vi "Controle_da_mesa_v3.vi"() -> ()   [LabVIEW 2017]
uses:
  <vilib>/Platform/TimedLoop/XDataNode/XDataNode.xnode
  <vilib>/Platform/TimedLoop/XDataNode/nitl_modes.ctl
  <vilib>/Platform/TimedLoop/XDataNode/XDNodeRunTimeDep.lvlib
  <vilib>/Platform/TimedLoop/XDataNode/wakeup.ctl
  <vilib>/Platform/TimedLoop/XDataNode/timing_clust.ctl
  <vilib>/Analysis/Matrix/NI_Matrix.lvlib
  <vilib>/Analysis/NI_AALPro.lvlib
  <vilib>/Analysis/NI_AALBase.lvlib
  <vilib>/Analysis/baseanly.llb/Real A x B.vi
  <vilib>/Analysis/Matrix/Numeric/Conversions/Matrix To Array - RM.vi
  <vilib>/Analysis/Matrix/Numeric/Conversions/Array To Matrix - RA.vi
  <vilib>/Analysis/Matrix/Numeric/Conversions/Array To Matrix - RA2.vi
  <vilib>/Analysis/_algsub.llb/Real PseudoInverse Matrix.vi
  <vilib>/rvi/interface/nirviCloseFPGA/nirviCloseFPGA.xnode
  <vilib>/rvi/interface/nirviMethod/nirviMethod.xnode
  <vilib>/rvi/interface/nirviMethod/StockFPGA_InlinedMethodWaitForSingleIRQ.vi
  <vilib>/FPGAPlugInAG/Dynamic/niLvFpga_WaitOnIrq_Dynamic.vi
  <vilib>/FPGAPlugInAG/Dynamic/niLvFpga_ReadFifo_Dynamic.vi
  <vilib>/rvi/errors/niLvFpgaMergeErrorWithErrorCode.vi
  <vilib>/FPGAPlugInAG/Dynamic/niLvFpga_AcknowledgeIrq_Dynamic.vi
  <vilib>/FPGAPlugInAG/Dynamic/niLvFpga_Close_Dynamic.vi
panel:
  out "Iteration Duration 2":i64
  out "error out 2":errorcluster
  out "error out":errorcluster
  in  "Stop_RT":bool
  out "Iteration Duration":i64
  out "INS":cluster{dbl[], sgl[]}[](graph)
  out "INS_R":bool
  out "CRC?":bool
  out "CRC Out":u16 format="%.0x"
  out "CRC_Input":u16 format="%x"
  out "LPI-X_R":sgl(slide)=-2.8742945e-05 scale=-6.0..6.0
  out "LPI-Y_R":sgl(slide)=-2.8742945e-05 scale=-6.0..6.0
  out "LPI-Z_R":sgl(slide)=-2.8742945e-05 scale=-6.0..6.0
  out "Longitude_R":sgl(slide)=-2.8742945e-05 scale=-180.0..180.0
  out "Altitude_R":sgl(slide)=-2.8742945e-05 scale=0.0..500.0
  out "Latitude_R":sgl(slide)=-2.8742945e-05 scale=-90.0..90.0
  out "Z_Accel_R":sgl(slide)=-2.8742945e-05 scale=-200.0..200.0
  out "X_Accel_R":sgl(slide)=-2.8742945e-05 scale=-200.0..200.0
  out "Y_Accel_R":sgl(slide)=-2.8742945e-05 scale=-200.0..200.0
  out "Z_Rate_R":sgl(slide)=-2.8742945e-05 scale=-300.0..300.0
  out "Y_ Rate_R":sgl(slide)=-2.8742945e-05 scale=-300.0..300.0
  out "X_Rate _R":sgl(slide)=-2.8742945e-05 scale=-300.0..300.0
  out "Yaw_R":sgl(slide)=-2.8742945e-05 scale=-180.0..180.0
  out "Pitch_R":sgl(slide)=-2.8742945e-05 scale=-90.0..90.0
  out "Roll_R":sgl(slide)=-2.8742945e-05 scale=-180.0..180.0
  out "Data Validity Time":u16[](array[numeric])
  out "Read String":string
  out "reserved 14":bool
  out "reserved 15":bool
  out "GC restarted 2":bool
  out "reserved 16":bool
  out "Init Align. M_Comp 2":bool
  out "Tick_Counter 2":u16
  out "Align_Word_Byte":bool[](array[boolean])
  out "GC_Counter 2":u32
  out "GC Align Counter (s) 2":bool[](array[boolean])
  out "Opp_Mode 2":string
  out "Fault_Code_HW 2":string
  out "ASE warning   2":bool
  out "Power warning 2":bool
  out "Motion Detection 2":bool
  out "RESERVED 4":bool
  out "RESERVED 5":bool
  out "RESERVED 6":bool
  out "Fault_Code 2":bool[](array[boolean])
  out "Operative_Mode 2":bool[](array[boolean])
  out "Op_Word_Byte":bool[](array[boolean])
  out "CRC_MSB 2":u8
  out "CRC_LSB 2":u8
  out "Status_Word_Byte":bool[](array[boolean])
  out "Data_Validity_Byte":bool[](array[boolean])
  out "outer previsto":dbl
  out "inner previsto":dbl
  in  "passo de predição":dbl=0.03 format="%#_13g"
  out "middle previsto":dbl
  out "Period":i64
  out "Middle":cluster{dbl[], dbl[]}[](graph)
  in  "Inicia seno":bool
  in  "Inner ON":bool
  in  "Middle ON":bool
  in  "Outer ON":bool
  in  "Amplitude Inner [deg]":dbl=1.0 format="%#_13g"
  in  "Amplitude Middle [deg]":dbl=1.0 format="%#_13g"
  in  "Amplitude Outer [deg]":dbl=1.0 format="%#_13g"
  in  "f inner [Hz]":dbl=1.0 format="%#_13g"
  in  "f middle [Hz]":dbl=1.0 format="%#_13g"
  in  "f outer [Hz]":dbl=1.0 format="%#_13g"
  out "spreadsheet string":string
  in  "UTC format":bool
  out "appended path":path
  out "concatenated string":string
  out "ACCEL":cluster{dbl, dbl, dbl} {"?" format="%1_6g"}
  out "RATE":cluster{dbl, dbl, dbl} {"?" format="%1_6g"}
  out "POS":cluster{dbl, dbl, dbl} {"?" format="%_6g"; "?" format="%#1_6g"}
  out "Tempo (s)":dbl
  out "string enviada para acutrol":string
  in  "Remote Host":string="192.168.53.1"
  in  "Para Controle da mesa":bool
  # "Atentar-se para que a posição inicial da mesa seja a mesma posição comandada. (Condições iniciais - Pos/Rate/Accel)"
  # "Monitor"
  # "Inner"
  # "Middle"
  # "Outer"
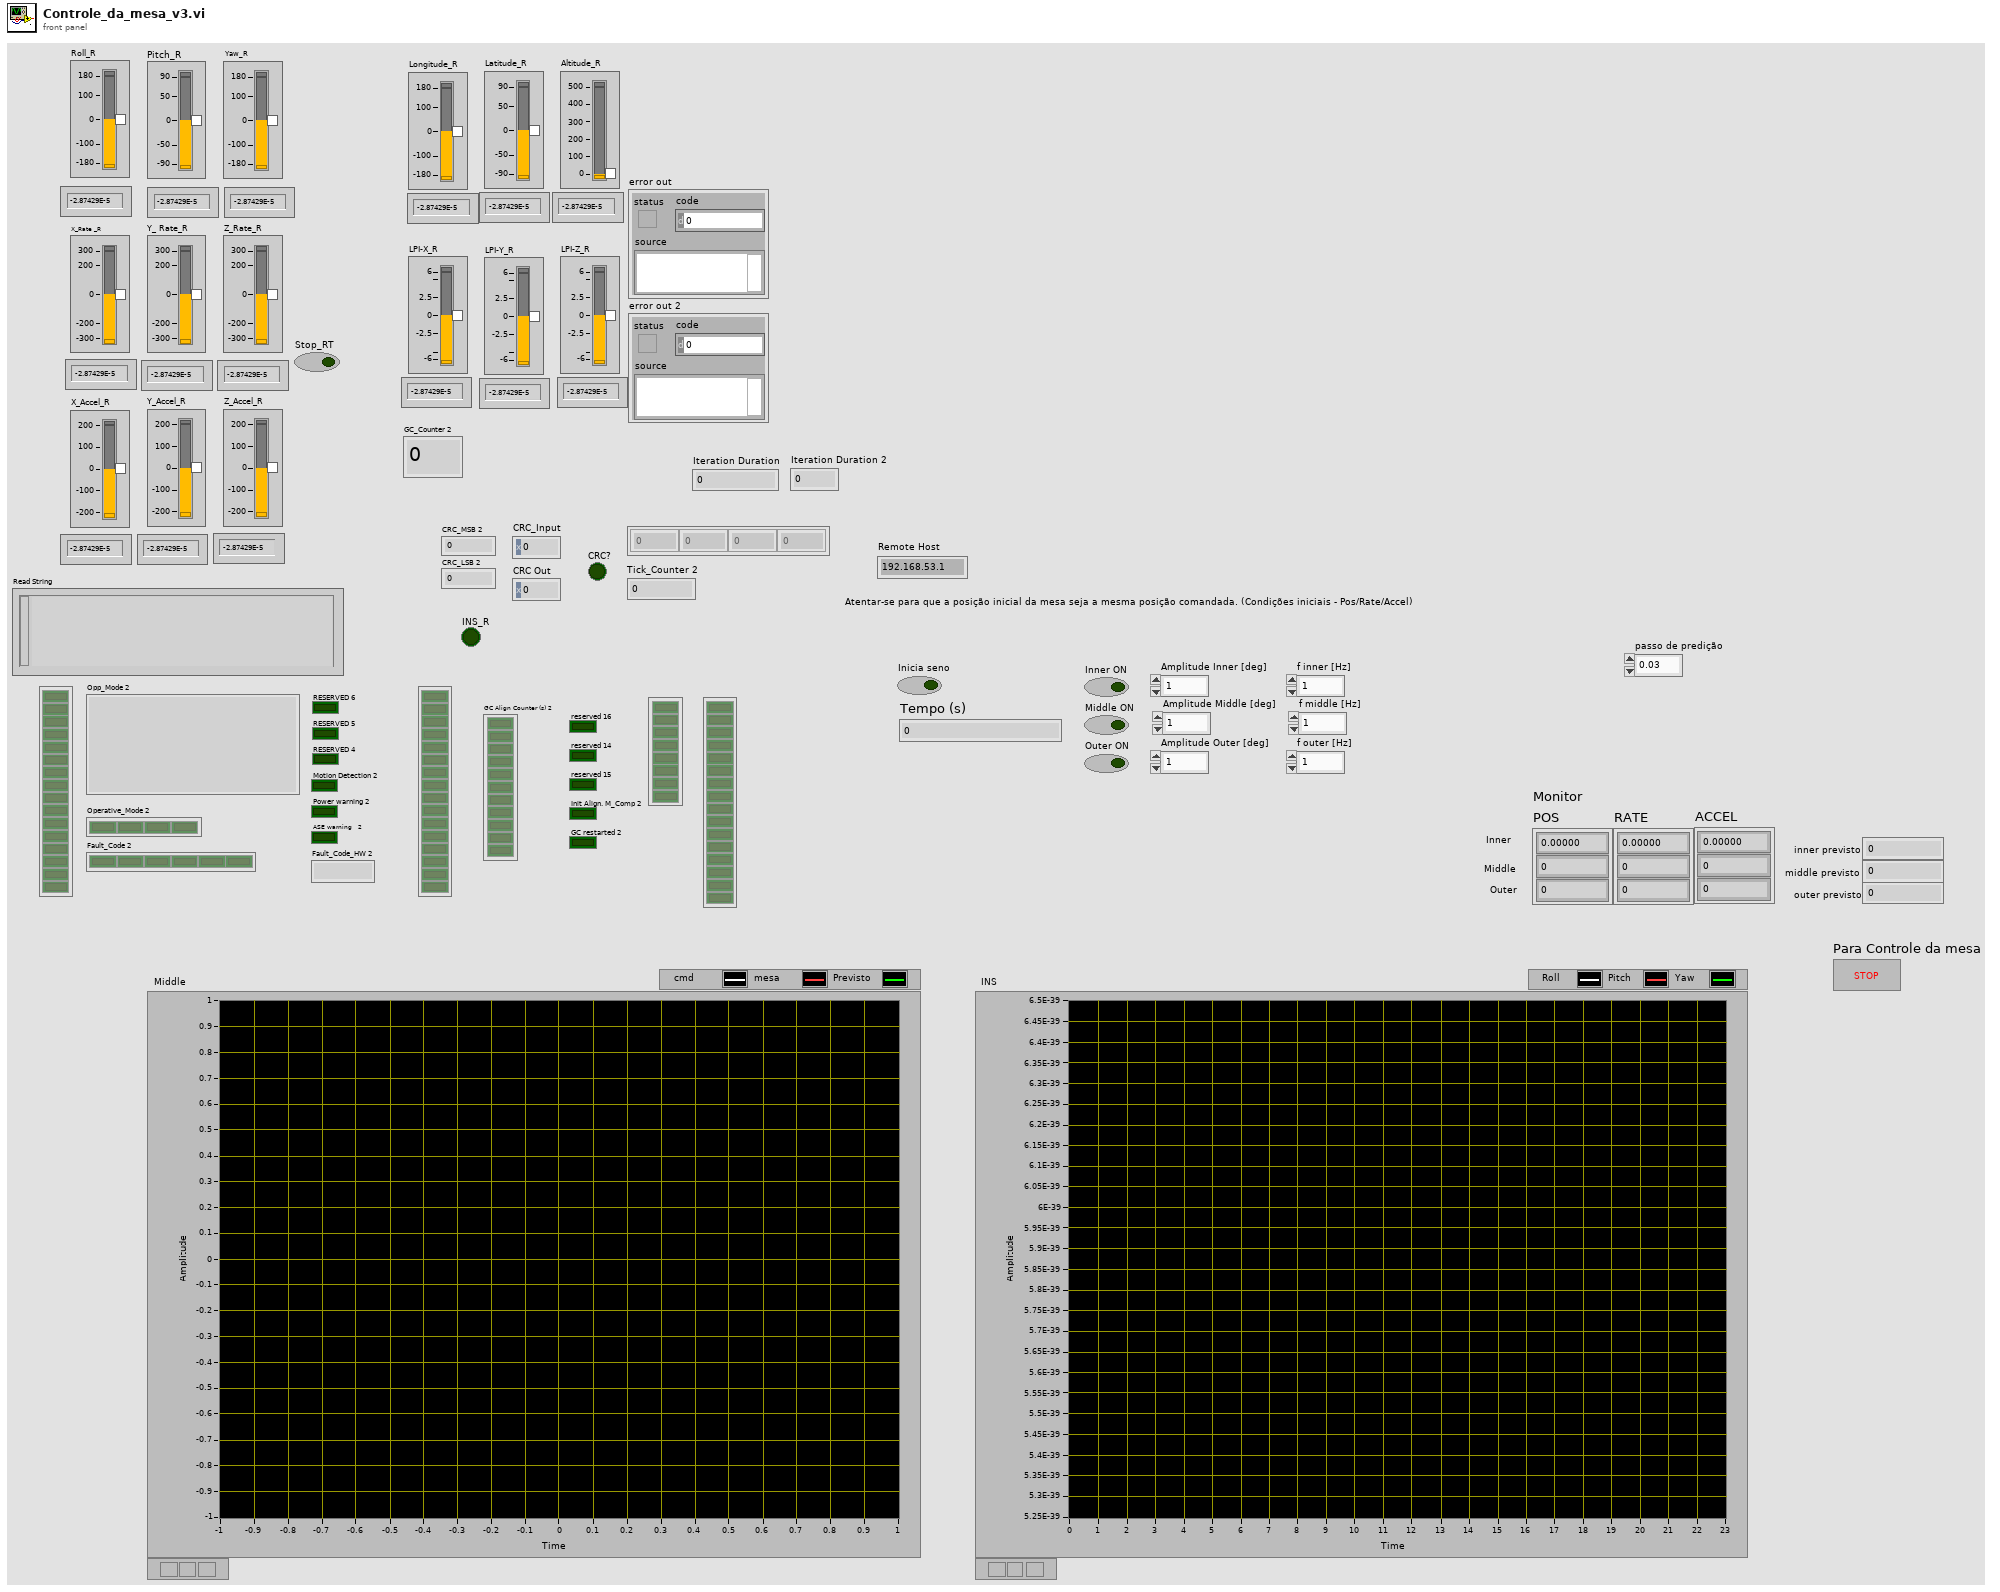
[diagram p1: front panel]
types:
  T1 = enum16{"open", "replace", "create", "open or create", "replace or create", "replace or create with confirmation"}
  T2 = typedef "XDNodeRunTimeDep.lvlib/timing_clust.ctl" = cluster{"Expected End [f-1]":u64, "Actual End [f-1]":u64, "Finished Late? [f-1]":bool, "Expected End [i-1]":u64, "Actual End [i-1]":u64, "Finished Late? [i-1]":bool, "Expected Start [i]":u64, "Actual Start [i]":u64, "Expected Start [f]":u64, "Actual Start [f]":u64, "Source Name":string, "Structure Name":string, "Period":i64, "Deadline":i64, "Offset":i64, "Start":i64, "Priority":i32, "Timeout":i32, "Mode":T3, "Wakeup Reason":T4, "Error":errorcluster, "Source Type":string, "Secondary Source Type":string, "Global End Time":u64, "Global Start Time":u64, "Frame Duration":u64, "Iteration Duration":u64, "Assigned CPU":i32, "I/O Scan Engine Mode":u32}
  T3 = typedef "XDNodeRunTimeDep.lvlib/nitl_modes.ctl" = enum32{"No Change", "Process missed periods, maintain original phase", "Discard missed periods, maintain original phase", "Process missed periods, ignore original phase", "Discard missed periods, ignore original phase"}
  T4 = typedef "XDNodeRunTimeDep.lvlib/wakeup.ctl" = enum32{"Normal", "Aborted", "Asynchronous wakeup", "Timing source error", "Timed loop error", "Timeout"}
  T5 = typedef "NI_Matrix.lvlib/RealMatrix.ctl" = dbl[][]
  T6 = cluster{"Roll_":sgl, "Pitch_":sgl, "Yaw_":sgl, "X_Rate":sgl, "Y_ Rate":sgl, "Z_Rate":sgl, "X_Accel":sgl, "Y_Accel":sgl, "Z_Accel":sgl, "Longitude":sgl, "Latitude":sgl, "Altitude":sgl, "LPI-X":sgl, "LPI-Y":sgl, "LPI-Z":sgl}
  T7 = cluster{"Op_Word_Byte":bool[], "Opp_Mode":string, "Operative_Mode":bool[], "RESERVED":bool, "RESERVED":bool, "RESERVED":bool, "Motion Detection":bool, "Power Warning":bool, "ASE Warning":bool, "Fault_Code":bool[], "Fault_Code_HW":string}
  T8 = cluster{"Align_Word_Byte":bool[], "GC Align Counter (s)":bool[], "GC_Counter":u32, "reserved":bool, "reserved":bool, "reserved":bool, "Init Align. M_Comp":bool, "GC restarted ":bool}
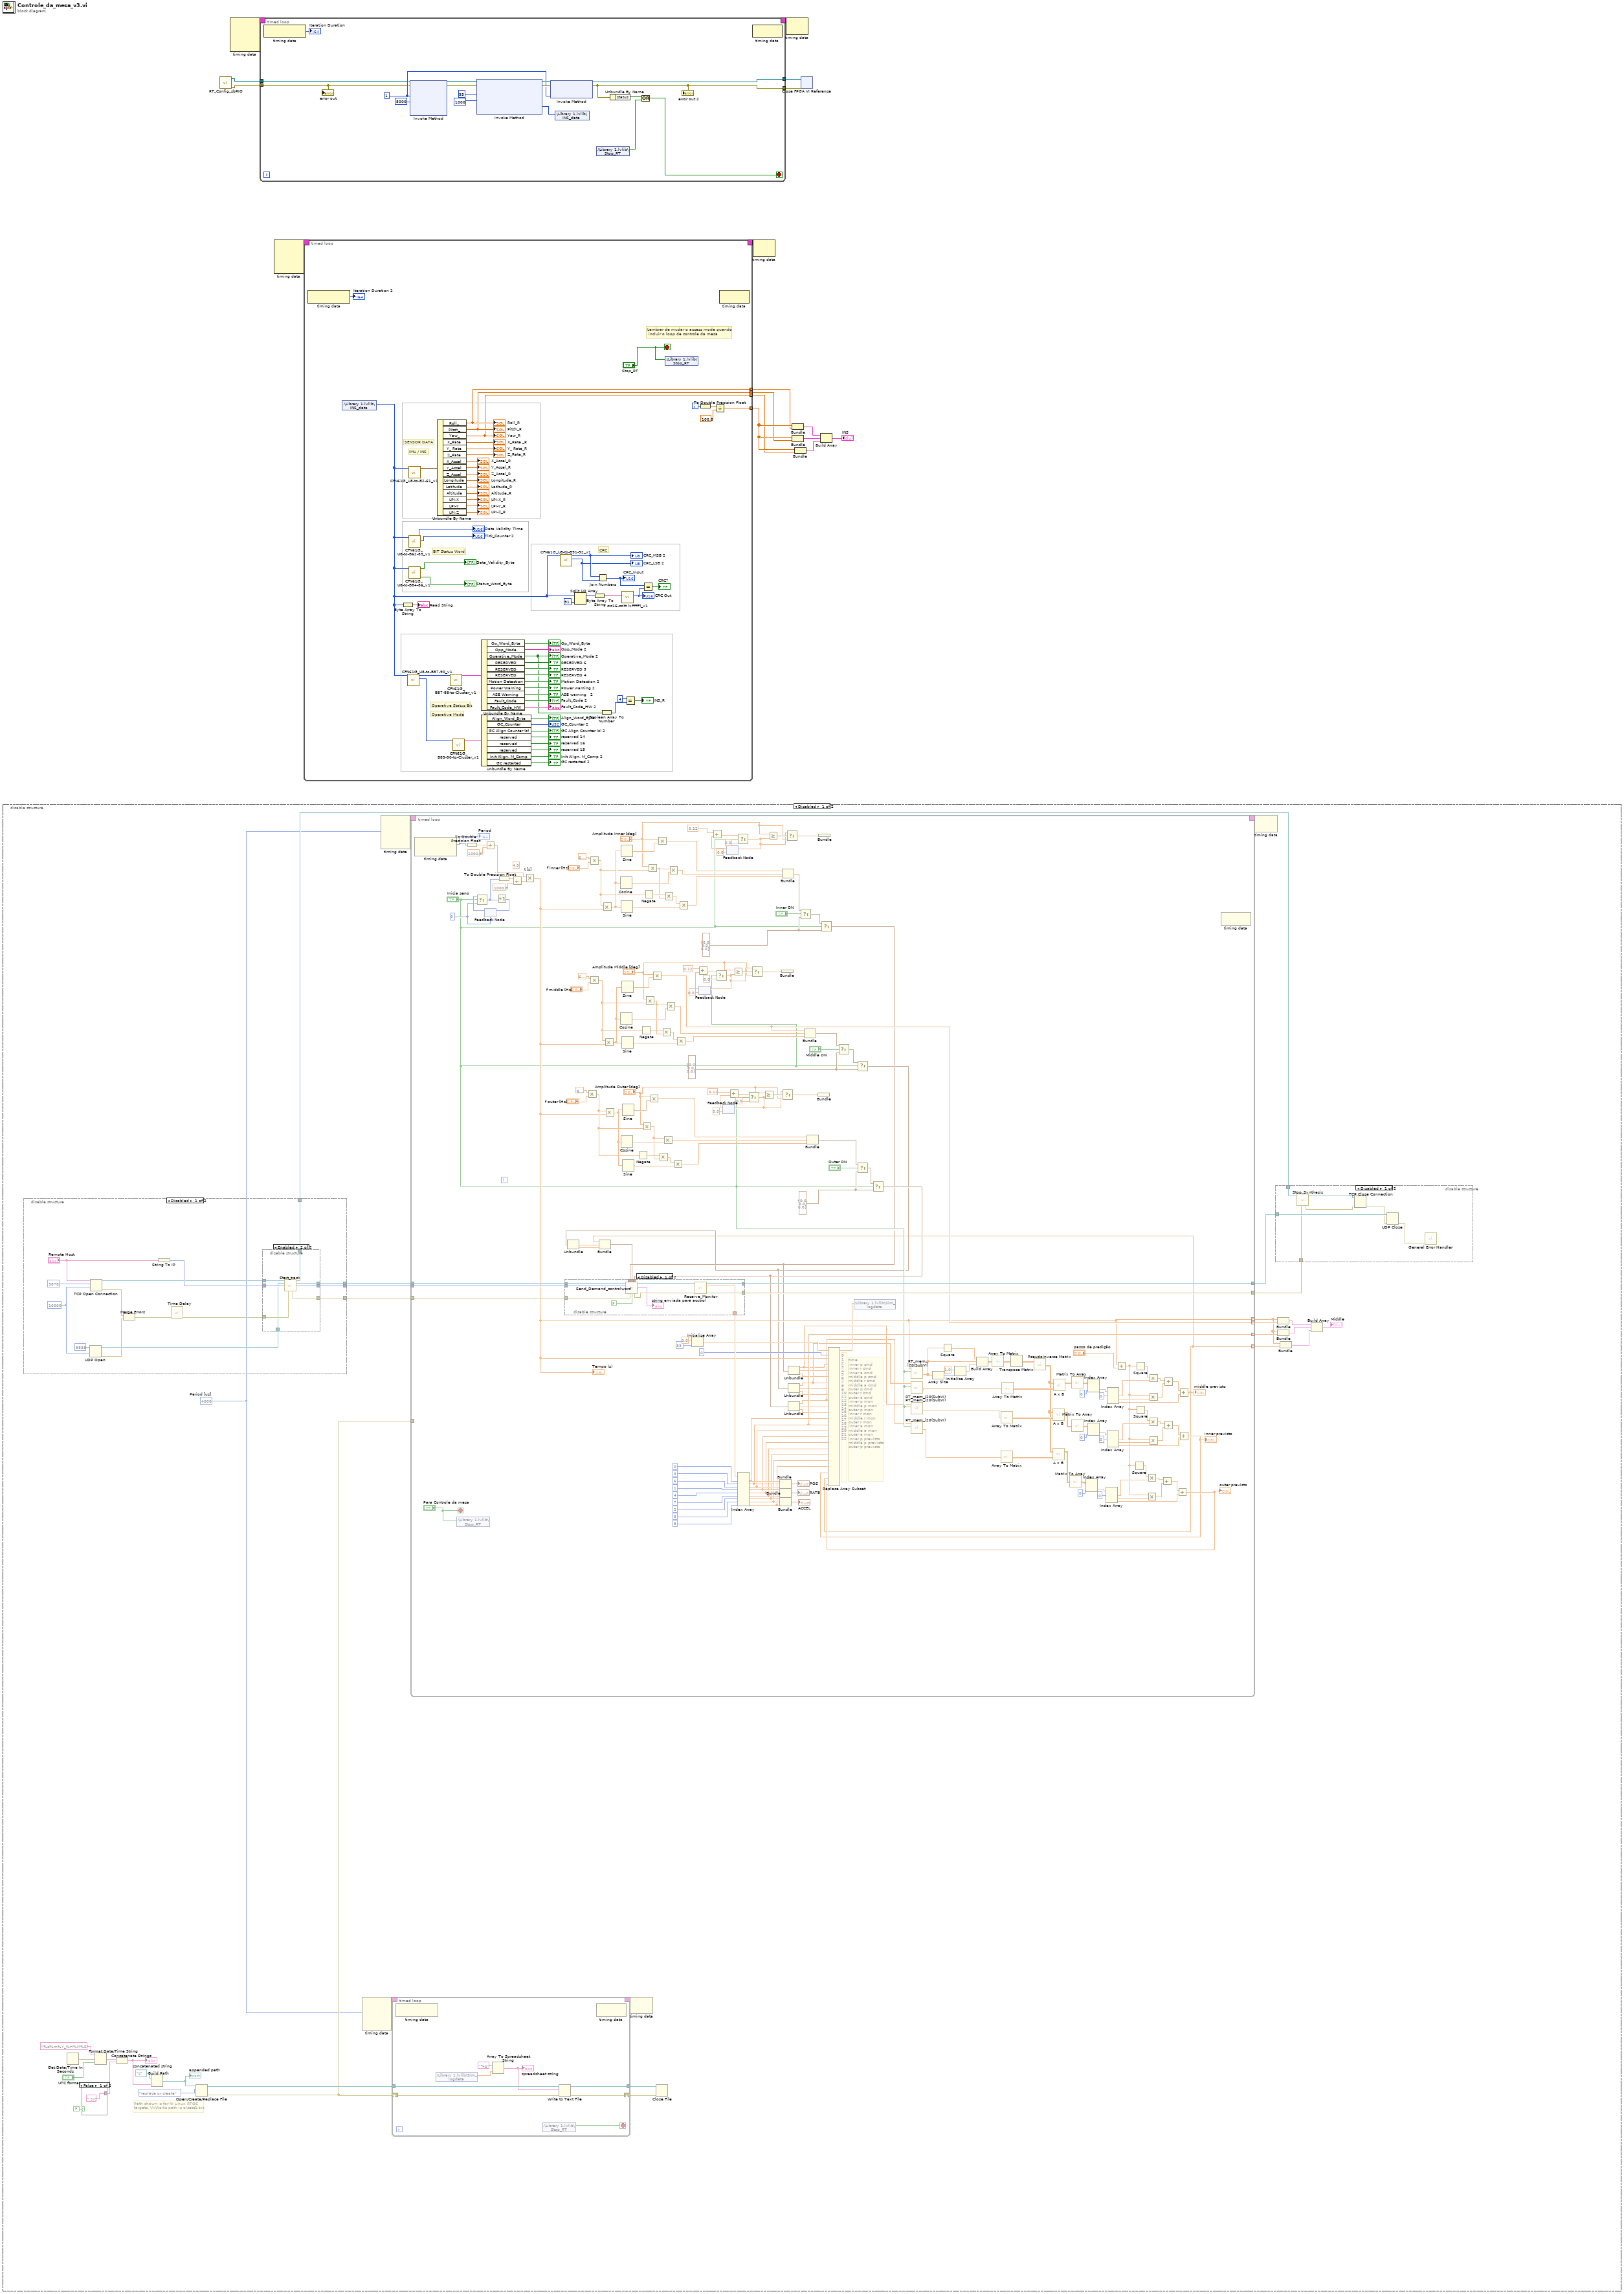
[diagram p0: block diagram]
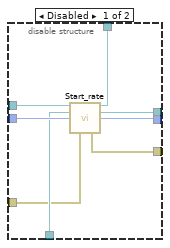
[diagram p3: hidden frame]
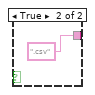
[diagram p6: hidden frame]
diagram:
  n1 = disable-structure shown="Disabled" {
    frame Disabled {
      w25 = i64 4000  # Period [us]
      # "Path shown is for NI Linux RTOS\ntargets. VxWorks path is c:\\test1.txt"
      n2 = disable-structure shown="Disabled" {
        disable-tunnel: [w67 _] -> w31
        disable-tunnel: [w66 _] -> w30
        disable-tunnel: [w65 _] -> w29
        disable-tunnel: [w64 _] -> w27
        frame Disabled {
          w58 = 10000 ("timeout ms (60000)")
          n3 = UDP Open(9:w58, 11:u16 9838 ("port")) -> (port=w70:refnum<k16>, 0:w57:errorcluster)  [unwired: 1 in, 3 out]
          n4 = TCP Open Connection(address="Remote Host", remote port or service name=u16 9878, timeout ms (60000)=w58) -> (connection ID=w69:refnum<k5>, error out=w59:errorcluster)  [unwired: 2 in]
          n5 = Merge Errors(w59, w57) -> (w62:errorcluster)
          n6 = String To IP(1:"Remote Host") -> (0:w71:u32)
          n7 = call "Time Delay"("error in (no error)"=w62) -> ("error out"=w68:errorcluster)  [unwired: 10 in]
          n8 = disable-structure shown="Enabled" {
            disable-tunnel: w71 -> [w79 w86]
            disable-tunnel: w70 -> [w78 w84]
            disable-tunnel: w69 -> [w77 w87]
            disable-tunnel: w68 -> [w76 w85]
            disable-tunnel: [w75 w82] -> w67
            disable-tunnel: [w74 w81] -> w66
            disable-tunnel: [w73 w80] -> w65
            disable-tunnel: [w72 w83] -> w64
            frame Disabled {
              n9 = call "Start_rate.vi"("TCP connection ID"=w77, "UDP connection ID"=w78, "IP address in"=w79, "error in"=w76) -> ("TCP connection ID out"=w72:refnum<k5>, "UDP connection ID out"=w75:refnum<k16>, "IP address out"=w74:u32, "error out"=w73:errorcluster)  [unwired: 7 in, 1 out]
            }
            frame Enabled {
              n10 = call "Start_track.vi"("TCP connection ID"=w87, "UDP connection ID"=w84, "IP address in"=w86, "error in"=w85) -> ("TCP connection ID out"=w83:refnum<k5>, "UDP connection ID out"=w82:refnum<k16>, "IP address out"=w81:u32, "error out"=w80:errorcluster)  [unwired: 7 in, 1 out]
            }
          }
        }
        frame Enabled {
        }
      }
      n11 = Get Date/Time In Seconds() -> (seconds since 1Jan1904=w35:timestamp)
      n12 = case shown="False" FALSE {
        tunnel: [".txt" ("string") ".csv" ("string")] -> w39
        frame False {
        }
        frame True {
        }
      }
      n13 = Format Date/Time String(time format string (%c)="%d%m%Y_%H%M%S", seconds (now)=w35, UTC format="UTC format") -> (date/time string=w34:string)
      n14 = Concatenate Strings(w34, w39) -> (w40:string)
      "concatenated string" <- w40
      n15 = Build Path(base path=path "c:/" ("file path (use dialog)"), name or relative path=w40) -> (appended path=w38:path)
      "appended path" <- w38
      n16 = Open/Create/Replace File(file path (use dialog)=w38, operation (0:open)=T1."replace or create") -> (refnum out=w43:refnum<file>, error out=w26:errorcluster)  [unwired: 4 in, 1 out]
      n17 = node-c288(w25) -> (w49:T2)  [unwired: 3 in]
      n18 = node-c288(w25) -> (w47:T2)  [unwired: 3 in]
      n19 = timed-loop {
        tunnel: w43 -> [w312]
        tunnel: [w311] -> w42
        timing: w49 -> [_]
        timing-out: [_] -> w48
        shift-right: [w305] -> w33
        shift-left: w26 -> [w306]
        stop <- w310 stop-if-true
        n20 = node-c288() -> ()  [unwired: 1 in, 1 out]
        n21 = shared-variable ".\\Library 1.lvlib\\Sim_logdata"() -> (w308:dbl[])  [unwired: 1 in, 1 out]
        n22 = Array To Spreadsheet String(array=w308, 3:"%g;" ("format string")) -> (spreadsheet string=w307:string)  [unwired: 1 in]
        "spreadsheet string" <- w307
        n23 = shared-variable ".\\Library 1.lvlib\\Stop_RT"() -> (w310:bool)  [unwired: 1 in, 1 out]
        n24 = Write to Text File(file (use dialog)=w312, text=w307, error in=w306) -> (refnum out=w311:refnum<file>, error out=w305:errorcluster)  [unwired: 1 in, 1 out]
        n25 = node-c288() -> ()  [unwired: 1 in, 1 out]
      }
      n26 = timed-loop {
        timing: w47 -> [_]
        timing-out: [_] -> w46
        tunnel: w31 -> [w280]
        tunnel: w30 -> [w279]
        tunnel: w29 -> [w278]
        tunnel: [w282] -> w28
        tunnel: [w281] -> w45
        tunnel: w26 -> [_]
        tunnel: [w138] -> w19 mode=indexing
        tunnel: [w155] -> w24 mode=indexing
        tunnel: [w173] -> w21 mode=indexing
        tunnel: [w88] -> w18 mode=indexing
        stop <- "Para Controle da mesa" stop-if-true
        w208 = cluster{dbl, dbl, dbl} {0.0, 0.0, 0.0} ("f")
        w212 = cluster{dbl, dbl, dbl} {0.0, 0.0, 0.0} ("f")
        w215 = cluster{dbl, dbl, dbl} {0.0, 0.0, 0.0} ("f")
        (unwired) 4.0 ("x")
        w257 = 0
        # "time\ninner p cmd\ninner r cmd\ninner a cmd\nmiddle p cmd\nmiddle r cmd\nmiddle a cmd\nouter p cmd\nouter r cmd\nouter a cmd\ninner p mon\nmiddle p mon\nouter p mon\ninner r mon\nmiddle r mon\nouter r mon\ninner a mon\nmiddle a mon\nouter a mon\ninner p previsto\nmiddle p previsto\nouter p previsto"
        # "0\n1\n2\n3\n4\n5\n6\n7\n8\n9\n10\n11\n12\n13\n14\n15\n16\n17\n18\n19\n20\n21\n22"
        n27 = node-c288() -> (w161:i64)  [unwired: 1 in, 1 out]
        "Period" <- w161
        n28 = shared-variable ".\\Library 1.lvlib\\Stop_RT"("Para Controle da mesa") -> ()  [unwired: 1 in, 1 out]
        n29 = To Double Precision Float(number=w161) -> (double precision float=w162:dbl)
        n30 = feedback #1(w257) -> (w258:i32)
        n31 = Select(t=w258, s="Inicia seno", f=w257) -> (s? t:f=w251:i32)
        n32 = Divide(x=w162, y=1000.0) -> (x/y=w160:dbl)
        n33 = Increment(x=w251) -> (x+1=w256:i32)
        n34 = feedback-in #1(w256) -> ()
        n35 = To Double Precision Float(number=w251) -> (double precision float=w252:dbl)
        n36 = Divide(x=w252, y=1000.0) -> (x/y=w250:dbl)
        n37 = Multiply "t [s]"(x=w160, y=w250) -> (x*y=w138:dbl)
        "Tempo (s)" <- w138
        n38 = Multiply(x=6.283185307179586, y="f outer [Hz]") -> (x*y=w218:dbl)
        n39 = Multiply(x=6.283185307179586, y="f inner [Hz]") -> (x*y=w242:dbl)
        n40 = Multiply(x=6.283185307179586, y="f middle [Hz]") -> (x*y=w219:dbl)
        n41 = Multiply(x=w242, y=w138) -> (x*y=w249:dbl)
        n42 = Multiply(x=w219, y=w138) -> (x*y=w223:dbl)
        n43 = Multiply(x=w218, y=w138) -> (x*y=w220:dbl)
        n44 = Cosine(x=w249) -> (cos(x)=w241:dbl)
        n45 = Cosine(x=w223) -> (cos(x)=w238:dbl)
        n46 = Cosine(x=w220) -> (cos(x)=w227:dbl)
        n47 = Sine(x=w249) -> (sin(x)=w243:dbl)
        n48 = Sine(x=w249) -> (sin(x)=w240:dbl)
        n49 = Sine(x=w223) -> (sin(x)=w237:dbl)
        n50 = Sine(x=w223) -> (sin(x)=w239:dbl)
        n51 = Sine(x=w220) -> (sin(x)=w228:dbl)
        n52 = Sine(x=w220) -> (sin(x)=w226:dbl)
        n53 = Negate(x=w218) -> (-x=w231:dbl)
        n54 = Negate(x=w219) -> (-x=w232:dbl)
        n55 = Multiply(x="Amplitude Outer [deg]", y=w218) -> (x*y=w230:dbl)
        n56 = Negate(x=w242) -> (-x=w248:dbl)
        n57 = Multiply(x="Amplitude Middle [deg]", y=w219) -> (x*y=w233:dbl)
        n58 = Multiply(x="Amplitude Inner [deg]", y=w242) -> (x*y=w247:dbl)
        n59 = Multiply(x="Amplitude Outer [deg]", y=w228) -> (x*y=w154:dbl)
        n60 = Multiply(x="Amplitude Middle [deg]", y=w237) -> (x*y=w155:dbl)
        n61 = Multiply(x="Amplitude Inner [deg]", y=w243) -> (x*y=w156:dbl)
        n62 = Multiply(x=w231, y=w230) -> (x*y=w229:dbl)
        n63 = Multiply(x=w232, y=w233) -> (x*y=w234:dbl)
        n64 = Multiply(x=w230, y=w227) -> (x*y=w171:dbl)
        n65 = Multiply(x=w248, y=w247) -> (x*y=w246:dbl)
        n66 = Multiply(x=w233, y=w238) -> (x*y=w235:dbl)
        n67 = Multiply(x=w247, y=w241) -> (x*y=w245:dbl)
        n68 = Multiply(x=w229, y=w226) -> (x*y=w170:dbl)
        n69 = Multiply(x=w234, y=w239) -> (x*y=w236:dbl)
        n70 = Multiply(x=w246, y=w240) -> (x*y=w244:dbl)
        n71 = Initialize Array(0.0 ("element"), 33 ("dimension size")) -> (w261:dbl[])
        n72 = feedback #2(0.0) -> (w184:dbl)
        n73 = Add(x=0.12, y=w184) -> (x+y=w185:dbl)
        n74 = Select(t=w185, s="Inicia seno", f=0.0) -> (s? t:f=w177:dbl)
        n75 = feedback-in #2(w177) -> ()
        n76 = feedback #3(0.0) -> (w182:dbl)
        n77 = feedback #4(0.0) -> (w180:dbl)
        n78 = Add(x=0.12, y=w180) -> (x+y=w181:dbl)
        n79 = Add(x=0.12, y=w182) -> (x+y=w183:dbl)
        n80 = Greater Or Equal?(x="Amplitude Middle [deg]", y=w177) -> (x >= y?=w194:bool)
        n81 = Select(t=w181, s="Inicia seno", f=0.0) -> (s? t:f=w179:dbl)
        n82 = feedback-in #4(w179) -> ()
        n83 = Select(t=w183, s="Inicia seno", f=0.0) -> (s? t:f=w175:dbl)
        n84 = feedback-in #3(w175) -> ()
        n85 = Select(t=w177, s=w194, f="Amplitude Middle [deg]") -> (s? t:f=w158:dbl)
        n86 = Greater Or Equal?(x="Amplitude Outer [deg]", y=w175) -> (x >= y?=w189:bool)
        n87 = Greater Or Equal?(x="Amplitude Inner [deg]", y=w179) -> (x >= y?=w195:bool)
        n88 = Bundle("Amplitude Middle [deg]"=w158) -> ()  [unwired: 1 in, 1 out]
        n89 = Bundle(w156, w245, w244) -> (w216:cluster{dbl, dbl, dbl})  [unwired: 1 in]
        n90 = Select(t=w175, s=w189, f="Amplitude Outer [deg]") -> (s? t:f=w157:dbl)
        n91 = Select(t=w179, s=w195, f="Amplitude Inner [deg]") -> (s? t:f=w159:dbl)
        n92 = Select(t=w216, s="Inner ON", f=w215) -> (s? t:f=w214:cluster{dbl, dbl, dbl})
        n93 = Bundle(w155, w235, w236) -> (w211:cluster{dbl, dbl, dbl})  [unwired: 1 in]
        n94 = Bundle(w154, w171, w170) -> (w207:cluster{dbl, dbl, dbl})  [unwired: 1 in]
        n95 = Bundle("Amplitude Outer [deg]"=w157) -> ()  [unwired: 1 in, 1 out]
        n96 = Bundle("Amplitude Inner [deg]"=w159) -> ()  [unwired: 1 in, 1 out]
        n97 = Select(t=w214, s="Inicia seno", f=w215) -> (s? t:f=w91:cluster{dbl, dbl, dbl})
        n98 = Unbundle(w91) -> (w127:dbl, w169:dbl, w168:dbl)
        n99 = Select(t=w211, s="Middle ON", f=w212) -> (s? t:f=w210:cluster{dbl, dbl, dbl})
        n100 = Select(t=w210, s="Inicia seno", f=w212) -> (s? t:f=w89:cluster{dbl, dbl, dbl})
        n101 = Unbundle(w89) -> (w93:dbl, w92:dbl)  [unwired: 1 out]
        n102 = Unbundle(w89) -> (w129:dbl, w167:dbl, w166:dbl)
        n103 = Select(t=w207, s="Outer ON", f=w208) -> (s? t:f=w206:cluster{dbl, dbl, dbl})
        n104 = Select(t=w206, s="Inicia seno", f=w208) -> (s? t:f=w172:cluster{dbl, dbl, dbl})
        n105 = Unbundle(w172) -> (w126:dbl, w165:dbl, w164:dbl)
        n106 = call "RT_mem_i20(SubVI).vi"("start"="Inicia seno", "In"=w138) -> ("in_vec"=w150:dbl[])  [unwired: 8 in, 1 out]
        n107 = call "RT_mem_i20(SubVI).vi"("start"="Inicia seno", "In"=w129) -> ("in_vec"=w130:dbl[])  [unwired: 8 in, 1 out]
        n108 = call "RT_mem_i20(SubVI).vi"("start"="Inicia seno", "In"=w127) -> ("in_vec"=w123:dbl[])  [unwired: 8 in, 1 out]
        n109 = call "RT_mem_i20(SubVI).vi"("start"="Inicia seno", "In"=w126) -> ("in_vec"=w122:dbl[])  [unwired: 8 in, 1 out]
        n110 = Array Size(array=w150) -> (size(s)=w153:i32)
        n111 = Square(x=w150) -> (x^2=w151:dbl[])
        n112 = Initialize Array(1.0 ("element"), w153) -> (w149:dbl[])
        n113 = Build Array(w151, w150, w149) -> (w147:dbl[][])
        n114 = call-poly <vilib>:"Array To Matrix.vi"("Real 2D Array"=w147) -> ("Real Matrix"=w148:T5)
        n115 = call-poly <vilib>:"Array To Matrix.vi"("Real 1D Array"=w123) -> ("Real Matrix (Column Vector)"=w125:T5)
        n116 = call-poly <vilib>:"Array To Matrix.vi"("Real 1D Array"=w122) -> ("Real Matrix (Column Vector)"=w124:T5)
        n117 = call-poly <vilib>:"Array To Matrix.vi"("Real 1D Array"=w130) -> ("Real Matrix (Column Vector)"=w145:T5)
        n118 = Transpose Matrix(1:w148) -> (0:w146:T5)
        n119 = call-poly <vilib>:"PseudoInverse Matrix.vi"("Input Matrix"=w146) -> ("PseudoInverse Matrix"=w99:T5)  [unwired: 1 in, 1 out]
        n120 = call-poly <vilib>:"A x B.vi"("B"=w125, "A"=w99) -> ("A x B"=w98:T5)  [unwired: 1 out]
        n121 = call-poly <vilib>:"A x B.vi"("B"=w124, "A"=w99) -> ("A x B"=w97:T5)  [unwired: 1 out]
        n122 = call-poly <vilib>:"A x B.vi"("B"=w145, "A"=w99) -> ("A x B"=w142:T5)  [unwired: 1 out]
        n123 = call-poly <vilib>:"Matrix To Array.vi"("Real Matrix"=w97) -> ("Real 2D Array"=w110:dbl[][])
        n124 = call-poly <vilib>:"Matrix To Array.vi"("Real Matrix"=w142) -> ("Real 2D Array"=w144:dbl[][])
        n125 = call-poly <vilib>:"Matrix To Array.vi"("Real Matrix"=w98) -> ("Real 2D Array"=w111:dbl[][])
        n126 = Index Array(array=w110, index (col)=0 ("index (row)")) -> (element=w108:dbl[])  [unwired: 1 in]
        n127 = Index Array(array=w144, index (col)=0 ("index (row)")) -> (element=w141:dbl[])  [unwired: 1 in]
        n128 = Index Array(array=w111, index (col)=0 ("index (row)")) -> (element=w113:dbl[])  [unwired: 1 in]
        n129 = Index Array(array=w108, index #1=0 ("index")) -> (element #1=w105:dbl, element #2=w103:dbl, element #3=w100:dbl)  [unwired: 2 in]
        n130 = Index Array(array=w141, index #1=0 ("index")) -> (element #1=w136:dbl, element #2=w134:dbl, element #3=w131:dbl)  [unwired: 2 in]
        n131 = Index Array(array=w113, index #1=0 ("index")) -> (element #1=w116:dbl, element #2=w118:dbl, element #3=w121:dbl)  [unwired: 2 in]
        n132 = Add(x=w138, y="passo de predição") -> (x+y=w96:dbl)
        n133 = Square(x=w96) -> (x^2=w106:dbl)
        n134 = Square(x=w96) -> (x^2=w137:dbl)
        n135 = Square(x=w96) -> (x^2=w115:dbl)
        n136 = Multiply(x=w106, y=w105) -> (x*y=w104:dbl)
        n137 = Multiply(x=w96, y=w103) -> (x*y=w102:dbl)
        n138 = Multiply(x=w137, y=w136) -> (x*y=w135:dbl)
        n139 = Multiply(x=w96, y=w134) -> (x*y=w133:dbl)
        n140 = Multiply(x=w115, y=w116) -> (x*y=w117:dbl)
        n141 = Multiply(x=w96, y=w118) -> (x*y=w119:dbl)
        n142 = Add(x=w104, y=w102) -> (x+y=w101:dbl)
        n143 = Add(x=w135, y=w133) -> (x+y=w132:dbl)
        n144 = Add(x=w117, y=w119) -> (x+y=w120:dbl)
        n145 = Add(x=w101, y=w100) -> (x+y=w95:dbl)
        "outer previsto" <- w95
        n146 = Add(x=w132, y=w131) -> (x+y=w88:dbl)
        "middle previsto" <- w88
        n147 = Bundle(w88, w93, w92) -> (w90:cluster{dbl, dbl, dbl})  [unwired: 1 in]
        n148 = disable-structure shown="Disabled" {
          disable-tunnel: [w295 _] -> w282
          disable-tunnel: [w294 _] -> w281
          disable-tunnel: w280 -> [w293 _]
          disable-tunnel: w279 -> [w292 _]
          disable-tunnel: w278 -> [w291 _]
          disable-tunnel: [w290 _] -> w269
          disable-tunnel: w172 -> [w289 _]
          disable-tunnel: w91 -> [w284 _]
          disable-tunnel: w90 -> [w283 _]
          frame Disabled {
            n149 = call "Send_Demand_controlword.vi"("UDP connection ID out"=w293, "Inner TRACK"=w284, "Middle TRACK"=w283, "Outer TRACK"=w289, "IP address in"=w292, "error in"=w291, "ReadOnly"=FALSE) -> ("UDP connection ID out"=w286:refnum<k16>, "concatenated string"=→"string enviada para acutrol":string, "error out"=w288:errorcluster)  [unwired: 5 in, 1 out]
            n150 = call "Receive_Monitor.vi"("UDP connection ID"=w286, "error out 2"=w288) -> ("UDP connection ID out"=w294:refnum<k16>, "MonitorBlock"=w290:dbl[], "error out"=w295:errorcluster)  [unwired: 11 in]
          }
          frame Enabled {
          }
        }
        n151 = Index Array(array=w269, index #1=0 ("index"), index #2=3 ("index"), index #3=6 ("index"), index #4=1 ("index"), index #5=4 ("index"), index #6=7 ("index"), index #7=2 ("index"), index #8=5 ("index"), index #9=8 ("index")) -> (element #1=w205:dbl, element #2=w173:dbl, element #3=w204:dbl, element #4=w203:dbl, element #5=w202:dbl, element #6=w201:dbl, element #7=w200:dbl, element #8=w199:dbl, element #9=w198:dbl)
        n152 = Bundle(w205, w173, w204) -> (→"POS":cluster{dbl, dbl, dbl})  [unwired: 1 in]
        n153 = Bundle(w203, w202, w201) -> (→"RATE":cluster{dbl, dbl, dbl})  [unwired: 1 in]
        n154 = Bundle(w200, w199, w198) -> (→"ACCEL":cluster{dbl, dbl, dbl})  [unwired: 1 in]
        n155 = Add(x=w120, y=w121) -> (x+y=w94:dbl)
        "inner previsto" <- w94
        n156 = Replace Array Subset(array=w261, new element #1=w138, index #1=0 ("index"), new element #2=w127, new element #3=w169, new element #4=w168, new element #5=w129, new element #6=w167, new element #7=w166, new element #8=w126, new element #9=w165, new element #10=w164, new element #11=w205, new element #12=w173, new element #13=w204, new element #14=w203, new element #15=w202, new element #16=w201, new element #17=w200, new element #18=w199, new element #19=w198, new element #20=w94, new element #21=w88, new element #22=w95) -> (w260:dbl[])  [unwired: 21 in]
        n157 = shared-variable ".\\Library 1.lvlib\\Sim_logdata"(w260) -> ()  [unwired: 1 in, 1 out]
        n158 = node-c288() -> ()  [unwired: 1 in, 1 out]
      }
      n159 = node-c288(w48) -> ()  [unwired: 1 out]
      n160 = Close File(refnum=w42, error in=w33) -> ()  [unwired: 2 out]
      n161 = node-c288(w46) -> ()  [unwired: 1 out]
      n162 = disable-structure shown="Disabled" {
        disable-tunnel: w45 -> [w56 _]
        disable-tunnel: w28 -> [w55 _]
        disable-tunnel: w27 -> [w54 _]
        frame Disabled {
          n163 = call "Stop_Synthesis.vi"("TCP connection ID"=w54, "error in"=w55) -> ("TCP connection ID out"=w52:refnum<k5>, "error out"=w51:errorcluster)  [unwired: 12 in]
          n164 = TCP Close Connection(connection ID=w52, error in (no error)=w51) -> (error out=w50:errorcluster)  [unwired: 1 in, 1 out]
          n165 = UDP Close(connection ID=w56, 8:w50) -> (error out=w53:errorcluster)  [unwired: 1 out]
          n166 = call <vilib>:"General Error Handler.vi"("error in (no error)"=w53) -> ()  [unwired: 2 in, 13 out]
        }
        frame Enabled {
        }
      }
      n167 = Bundle(w19, w24) -> (w23:cluster{dbl[], dbl[]})  [unwired: 1 in]
      n168 = Bundle(w19, w21) -> (w22:cluster{dbl[], dbl[]})  [unwired: 1 in]
      n169 = Bundle(w19, w18) -> (w17:cluster{dbl[], dbl[]})  [unwired: 1 in]
      n170 = Build Array(w23, w22, w17) -> (→"Middle":cluster{dbl[], dbl[]}[])
    }
    frame Enabled {
    }
  }
  n171 = call "RT_Config_sbRIO.vi"() -> ("error out"=w15:errorcluster, "FPGA VI Reference Out"=w16:refnum<k20>)  [unwired: 10 in]
  n172 = node-c288() -> (w12:T2)  [unwired: 4 in]
  n173 = timed-loop {
    tunnel: w16 -> [w324]
    tunnel: w15 -> [w323]
    tunnel: [w322] -> w14
    tunnel: [w321] -> w13
    timing: w12 -> [_]
    timing-out: [_] -> w11
    stop <- w320 stop-if-true
    w327 = 1 ("IRQ Number(s)")
    n174 = node-c288() -> (→"Iteration Duration":i64)  [unwired: 1 in]
    n175 = xnode "Invoke Method"("FPGA VI Reference In"=w324, "error in"=w323, "IRQ Number(s)"=w327, "Timeout (ms)"=5000) -> ("FPGA VI Reference Out"=w333:refnum<k20>, "error out"=w332:errorcluster)  [unwired: 2 out]
    n176 = xnode "Invoke Method"("FPGA VI Reference In"=w333, "error in"=w332, "Number of Elements"=u32 93, "Timeout (ms)"=1000) -> ("FPGA VI Reference Out"=w331:refnum<k20>, "error out"=w330:errorcluster, "Data"=w325:u8[])  [unwired: 1 out]
    n177 = xnode "Invoke Method"("FPGA VI Reference In"=w331, "error in"=w330, "IRQ Number(s)"=w327) -> ("FPGA VI Reference Out"=w322:refnum<k20>, "error out"=w321:errorcluster)
    "error out 2" <- w321
    n178 = shared-variable ".\\Library 1.lvlib\\INS_data"(w325) -> ()  [unwired: 1 in, 1 out]
    n179 = shared-variable ".\\Library 1.lvlib\\Stop_RT"() -> (w326:bool)  [unwired: 1 in, 1 out]
    n180 = Unbundle By Name(w321) -> ("status"=w335:bool)
    n181 = Or(x=w335, y=w326) -> (x .or. y?=w320:bool)
    n182 = node-c288() -> ()  [unwired: 1 in, 1 out]
    "error out" <- w323
  }
  n183 = node-c288() -> (w10:T2)  [unwired: 4 in]
  n184 = timed-loop {
    timing: w10 -> [_]
    timing-out: [_] -> w9
    tunnel: [w345] -> w5 mode=indexing
    tunnel: [w344] -> w4 mode=indexing
    tunnel: [w343] -> w3 mode=indexing
    tunnel: [w342] -> w2 mode=indexing
    i -> [w348]
    stop <- "Stop_RT" stop-if-true
    # "Lembrar de mudar o access mode quando\n incluir o loop de controle da mesa"
    # "Operative Mode"
    # "CRC"
    # "Operative Status Bit"
    # "BIT Status Word"
    # "IMU / INS"
    # "SENSOR DATA"
    n185 = node-c288() -> (→"Iteration Duration 2":i64)  [unwired: 1 in]
    n186 = shared-variable ".\\Library 1.lvlib\\INS_data"() -> (w341:u8[])  [unwired: 1 in, 1 out]
    n187 = Byte Array To String(unsigned byte array=w341) -> (string=→"Read String":string)
    n188 = call "CFN61G_U8-to-B87-90_v1.vi"("U8_Input"=w341) -> ("Align_Word"=w389:u16, "Op_Word"=w378:u16)  [unwired: 9 in]
    n189 = call "CFN61G_U8-to-B2-61_v1.vi"("U8_Input"=w341) -> ("Output_Cluster"=w367:T6)  [unwired: 10 in]
    n190 = call "CFN61G_U8-to-B62-83_v1.vi"("U8_Input"=w341) -> ("Tick_Counter"=→"Tick_Counter 2":u16, "Data Validity Time"=→"Data Validity Time":u16[])  [unwired: 8 in, 1 out]
    n191 = call "CFN61G_U8-to-B84-86_v1.vi"("U8_Input"=w341) -> ("Status_Word_Byte"=→"Status_Word_Byte":bool[], "Data_Validity_Byte"=→"Data_Validity_Byte":bool[])  [unwired: 7 in, 2 out]
    n192 = Unbundle By Name(w367) -> ("Roll_"=w344:sgl, "Pitch_"=w343:sgl, "Yaw_"=w342:sgl, "X_Rate"=→"X_Rate _R":sgl, "Y_ Rate"=→"Y_ Rate_R":sgl, "Z_Rate"=→"Z_Rate_R":sgl, "X_Accel"=→"X_Accel_R":sgl, "Y_Accel"=→"Y_Accel_R":sgl, "Z_Accel"=→"Z_Accel_R":sgl, "Longitude"=→"Longitude_R":sgl, "Latitude"=→"Latitude_R":sgl, "Altitude"=→"Altitude_R":sgl, "LPI-X"=→"LPI-X_R":sgl, "LPI-Y"=→"LPI-Y_R":sgl, "LPI-Z"=→"LPI-Z_R":sgl)
    "Roll_R" <- w344
    "Pitch_R" <- w343
    "Yaw_R" <- w342
    n193 = call "CFN61G_B87-88-to-Cluster_v1.vi"("Op_Word"=w378) -> ("output cluster"=w377:T7)  [unwired: 10 in]
    n194 = call "CFN61G_B89-90-to-Cluster_v1.vi"("Align_Word"=w389) -> ("Cluster"=w376:T8)  [unwired: 10 in]
    n195 = Unbundle By Name(w377) -> ("Op_Word_Byte"=→"Op_Word_Byte":bool[], "Opp_Mode"=→"Opp_Mode 2":string, "Operative_Mode"=w355:bool[], "RESERVED"=→"RESERVED 6":bool, "RESERVED"=→"RESERVED 5":bool, "RESERVED"=→"RESERVED 4":bool, "Motion Detection"=→"Motion Detection 2":bool, "Power Warning"=→"Power warning 2":bool, "ASE Warning"=→"ASE warning   2":bool, "Fault_Code"=→"Fault_Code 2":bool[], "Fault_Code_HW"=→"Fault_Code_HW 2":string)
    "Operative_Mode 2" <- w355
    n196 = Unbundle By Name(w376) -> ("Align_Word_Byte"=→"Align_Word_Byte":bool[], "GC_Counter"=→"GC_Counter 2":u32, "GC Align Counter (s)"=→"GC Align Counter (s) 2":bool[], "reserved"=→"reserved 14":bool, "reserved"=→"reserved 16":bool, "reserved"=→"reserved 15":bool, "Init Align. M_Comp"=→"Init Align. M_Comp 2":bool, "GC restarted"=→"GC restarted 2":bool)
    n197 = call "CFN61G_U8-to-B91-92_v1.vi"("U8_Injput"=w341) -> ("CRC_LSB"=w359:u8, "CRC_MSB"=w360:u8)  [unwired: 9 in]
    "CRC_LSB 2" <- w359
    "CRC_MSB 2" <- w360
    n198 = Split 1D Array(array=w341, index=91) -> (first subarray=w365:u8[])  [unwired: 1 out]
    n199 = Byte Array To String(unsigned byte array=w365) -> (string=w364:string)
    n200 = Join Numbers(hi=w360, lo=w359) -> ((hi.lo)=w363:u16)
    "CRC_Input" <- w363
    n201 = Boolean Array To Number(Boolean array=w355) -> (number=w354:u32)
    n202 = call "crc16-ccitt (xFFFF)_v1.vi"("Message"=w364) -> ("CRC"=w362:u16)  [unwired: 9 in, 1 out]
    "CRC Out" <- w362
    n203 = Equal?(x=u32 4, y=w354) -> (x = y?=→"INS_R":bool)
    n204 = Equal?(x=w363, y=w362) -> (x = y?=→"CRC?":bool)
    n205 = shared-variable ".\\Library 1.lvlib\\Stop_RT"("Stop_RT") -> ()  [unwired: 1 in, 1 out]
    n206 = To Double Precision Float(number=w348) -> (double precision float=w347:dbl)
    n207 = Divide(x=w347, y=100.0) -> (x/y=w345:dbl)
    n208 = node-c288() -> ()  [unwired: 1 in, 1 out]
  }
  n209 = node-c288(w9) -> ()  [unwired: 1 out]
  n210 = node-c288(w11) -> ()  [unwired: 1 out]
  n211 = Bundle(w5, w4) -> (w8:cluster{dbl[], sgl[]})  [unwired: 1 in]
  n212 = Bundle(w5, w3) -> (w7:cluster{dbl[], sgl[]})  [unwired: 1 in]
  n213 = Bundle(w5, w2) -> (w6:cluster{dbl[], sgl[]})  [unwired: 1 in]
  n214 = xnode "Close FPGA VI Reference"("FPGA VI Reference In"=w14, "error in"=w13) -> ()  [unwired: 1 out]
  n215 = Build Array(w8, w7, w6) -> (→"INS":cluster{dbl[], sgl[]}[])
